vi "lab3.vi"() -> ()   [LabVIEW 2020]
uses:
  4ff7459a-8349-4664-9fea-9f1d000a3dcd.vi
  69688eac-17de-477d-92d3-75e518164099.vi
  <vilib>/Array/Sort 2D Array - Pop Stack.vi
  <vilib>/Array/Sort 2D Array - Push Stack.vi
  69688eac-17de-477d-92d3-75e518164099.vi/269d4b3b-47f5-49e3-8884-44851e4dd9d5.vi
  69688eac-17de-477d-92d3-75e518164099.vi/6d99389c-673d-4efb-bf33-19b32bcf4cf8.vi
  <vilib>/Comparison/Less/Less Functor/Less Functor.lvclass
panel:
  out "Stop boolean":bool
  in  "stop":bool
  in  "Iteration delay":u32
  out "i":i32
  out "Max values graph 10x":dbl[](graph)
  out "Max values graph":dbl[](graph)
  out "Max waveform":dbl(graph)
  out "sorted 2D array":dbl[][](array[numeric])
  out "Array with sorted rows":dbl[][](array[numeric])
  out "Generated array":dbl[][](array[numeric])
  out "Last generated value (0 to 1)":dbl
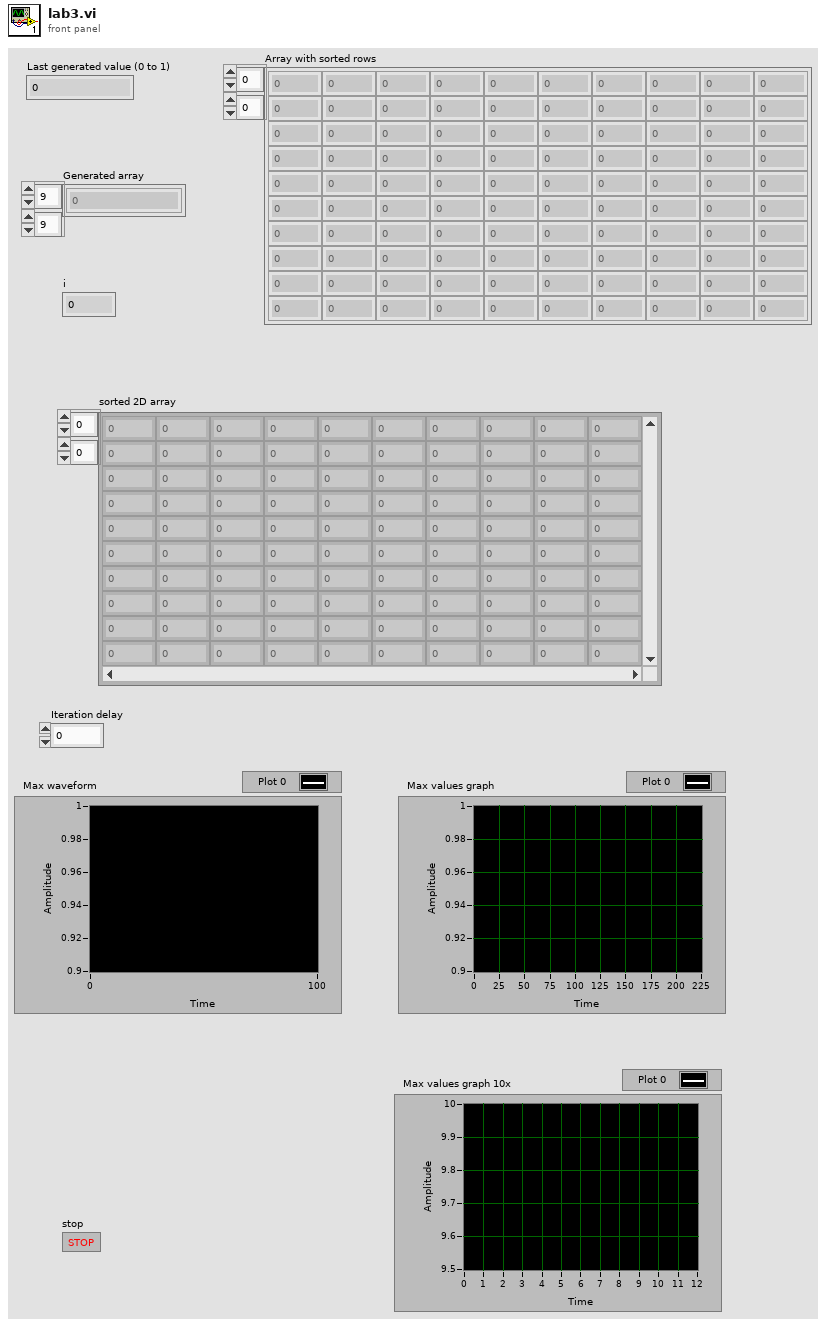
[diagram p1: front panel]
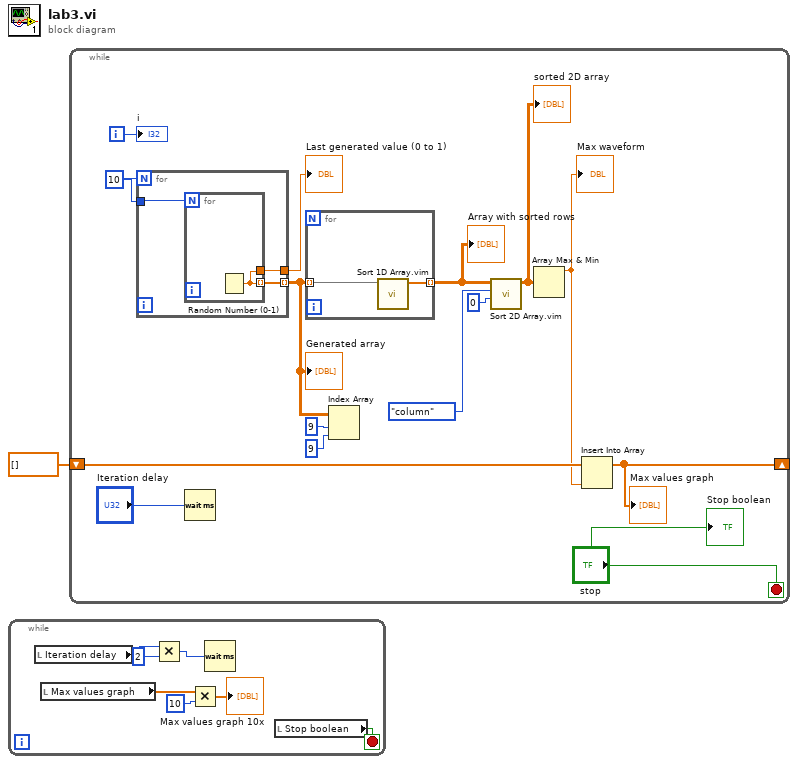
[diagram p0: block diagram]
diagram:
  n1 = while {
    stop <- w5 stop-if-true
    n2 = local read "Iteration delay"() -> (w4:u32)
    n3 = local read "Max values graph"() -> (w8:dbl[])
    n4 = Multiply(x=w4, y=u32 2) -> (x*y=w3:u32)
    n5 = Multiply(x=w8, y=10) -> (x*y=→"Max values graph 10x":dbl[])
    n6 = Wait (ms)(milliseconds to wait=w3) -> ()  [unwired: 1 out]
    n7 = local read "Stop boolean"() -> (w5:bool)
  }
  n8 = while {
    shift-right: [w12] -> _
    shift-left: dbl[] [] -> [w14]
    i -> [w11]
    stop <- "stop" stop-if-true
    w23 = 10
    n9 = for {
      N: w23 -> [_]
      tunnel: w23 -> [w28]
      tunnel: [w27] -> w22
      tunnel: [w26] -> w19 mode=indexing
      n10 = for {
        N: w28 -> [_]
        tunnel: [w29] -> w27
        tunnel: [w29] -> w26 mode=indexing
        n11 = Random Number (0-1)() -> (number: 0 to 1=w29:dbl)
      }
    }
    "Last generated value (0 to 1)" <- w22
    "Generated array" <- w19
    n12 = Wait (ms)(milliseconds to wait="Iteration delay") -> ()  [unwired: 1 out]
    n13 = for {
      tunnel: w19 -> [w25] mode=indexing
      tunnel: [w24] -> w16 mode=indexing
      n14 = call "Sort 1D Array.vim"("unsorted array"=w25) -> ("sorted array"=w24:dbl[])  [unwired: 10 in]
    }
    "Array with sorted rows" <- w16
    n15 = Index Array(array=w19, index (row)=9, index (col)=9 ("disabled index (col)")) -> ()  [unwired: 1 out]
    n16 = call "Sort 2D Array.vim"("index"=0, "dimension to index (column)"=enum16{"column", "row"}."column", "2D array"=w16) -> ("sorted 2D array"=w15:dbl[][])  [unwired: 7 in, 1 out]
    "sorted 2D array" <- w15
    n17 = Array Max & Min(array=w15) -> (max value=w13:dbl)  [unwired: 3 out]
    "Max waveform" <- w13
    n18 = Insert Into Array(array=w14, new element=w13) -> (w12:dbl[])  [unwired: 1 in]
    "Max values graph" <- w12
    "i" <- w11
    "Stop boolean" <- "stop"
  }
